vi "Dequeue.vi"(8 "error in (no error)":errorcluster) -> (0 "error out":errorcluster, 2 "Data":variant, 3 "State":T1)   [LabVIEW 2018, in "User Console.lvlib"]
doc: "Dequeues elements from the module queue."
uses:
  User Console.lvlib
  ctl/Module State--enum.ctl
  Module Queue Actions.ctl
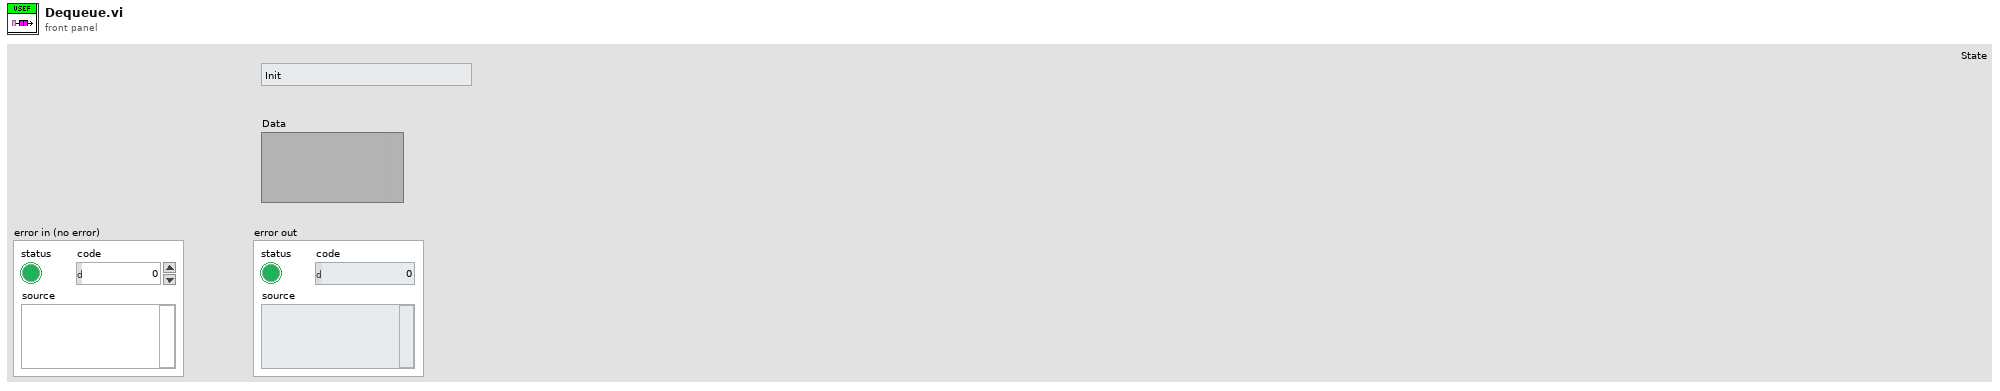
[diagram p1: front panel]
types:
  T1 = typedef "User Console.lvlib/Module State--enum.ctl" = enum16{"Init", "Error", "Idle", "Close", "Transaction Button Pressed: Which?", "Balance Inquiry Pressed", "Desposit Pressed", "Withdrawal Pressed", "Fast Cash Pressed", "New Transaction Pressed", "Terminate Session Pressed", "Card Reader Pressed", "Keypad Button Pressed", "Update Keypad Screen", "Enable/disable controls", "Card reader: On?"}
  T2 = typedef "User Console.lvlib/Module Queue Actions.ctl" = enum16{"Create", "Get", "Destroy"}
  T3 = typedef "User Console.lvlib/Module Message--cluster.ctl" = cluster{"State":T1, "Data":variant}
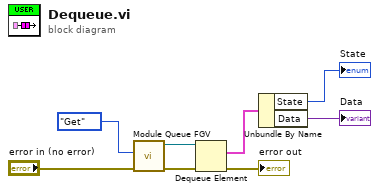
[diagram p0: block diagram]
diagram:
  n1 = call "Module Queue FGV.vi"("Error in"="error in (no error)", "Module Queue Actions"=Module_Queue_Actions."Get") -> ("error out"=w5:errorcluster, "Queue out"=w6:refnum<queue>)  [unwired: 8 in]
  n2 = Dequeue Element(queue=w6, error in (no error)=w5) -> (element=w4:T3, error out=→"error out":errorcluster)  [unwired: 1 in, 2 out]
  n3 = Unbundle By Name(w4) -> ("State"=→"State":T1, "Data"=→"Data":variant)
